vi "Read Display Values.vi"(0 "VISA resource name":refnum<visa-resource-name>, 2 "Communication Address (0)":i16 max=254 format="%x", 11 "error in (no error)":errorcluster) -> (4 "VISA resource name out":refnum<visa-resource-name>, 6 "Terminal Output Current":dbl format="%#.2g", 8 "Terminal Output Voltage":dbl format="%#.2g", 15 "error out":errorcluster)   [LabVIEW 2019, in "BK Precision 178XB Series.lvlib"]
doc: "This VI reads the voltage and current value at the terminal output of the power supply. It is the same value that is displayed on the instrument when the supply output is on."
uses:
  BK Precision 178XB Series.lvlib
panel:
  # "(c) 2009 B&K PRECISION CORPORATION.  ALL RIGHTS RESERVED."
  # "A"
  # "V"
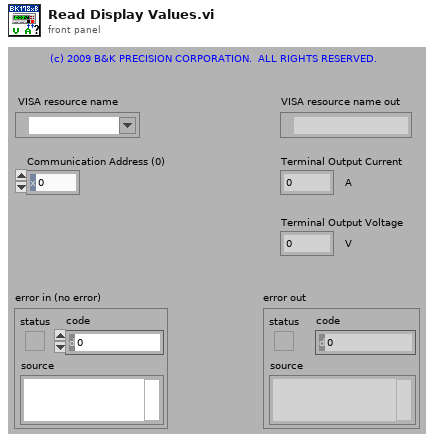
[diagram p1: front panel]
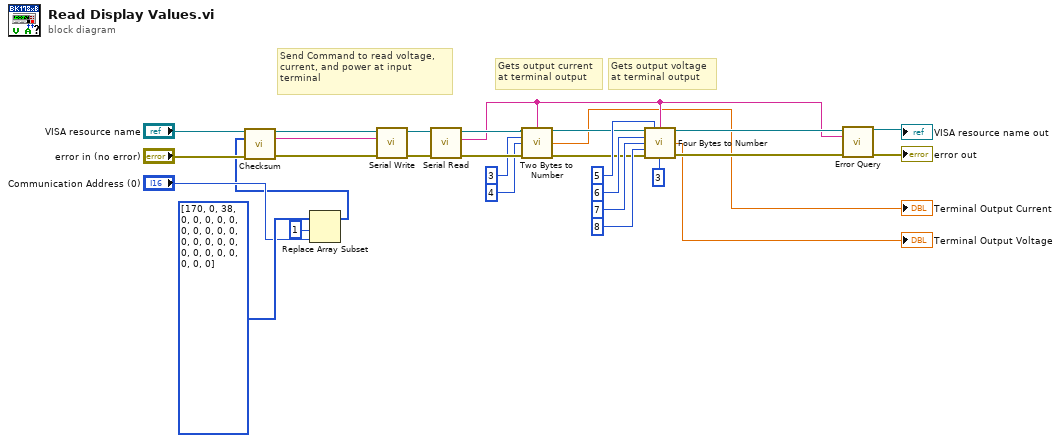
[diagram p0: block diagram]
diagram:
  # "Gets output voltage\nat terminal output"
  # "Gets output current\nat terminal output"
  # "Send Command to read voltage,\ncurrent, and power at input\nterminal"
  n1 = Replace Array Subset(array=i16[] [170, 0, 38, 0, 0, 0, 0, 0, 0, 0, 0, 0, 0, 0, 0, 0, 0, 0, 0, 0, 0, 0, 0, 0, 0, 0], new element="Communication Address (0)", index=1) -> (w1:i16[])
  n2 = call "Checksum.vi"("VISA resource name"="VISA resource name", "Command Frame Array"=w1, "error in (no error)"="error in (no error)") -> ("VISA resource name out"=w22:refnum<visa-resource-name>, "Output String"=w21:string, "error out"=w23:errorcluster)  [unwired: 8 in, 2 out]
  n3 = call "Serial Write.vi"("error in (no error)"=w23, "Input Command Frame"=w21, "VISA resource name"=w22) -> ("error out"=w27:errorcluster, "VISA resource name out"=w26:refnum<visa-resource-name>)  [unwired: 6 in, 1 out]
  n4 = call "Serial Read.vi"("error in (no error)"=w27, "VISA resource name"=w26) -> ("error out"=w16:errorcluster, "Read Buffer"=w7:string, "VISA resource name out"=w15:refnum<visa-resource-name>)  [unwired: 7 in]
  n5 = call "Two Bytes to Number.vi"("VISA resource name"=w15, "Input Command Frame"=w7, "Index 0 (3)"=3, "Index 1 (4)"=4, "error in (no error)"=w16) -> ("VISA resource name out"=w14:refnum<visa-resource-name>, "Numerical Value"=→"Terminal Output Current":dbl, "error out"=w13:errorcluster)  [unwired: 8 in]
  n6 = call "Four Bytes to Number.vi"("VISA resource name"=w14, "Index 0 (3)"=5, "Input Command Frame"=w7, "Index 1 (4)"=6, "Index 2 (5)"=7, "Index 3 (6)"=8, "error in (no error)"=w13, "Decimal Offset (3)"=3) -> ("VISA resource name out"=w8:refnum<visa-resource-name>, "Numerical Value"=→"Terminal Output Voltage":dbl, "error out"=w9:errorcluster)  [unwired: 5 in]
  n7 = call "Error Query.vi"("VISA resource name"=w8, "Input Read Buffer 1"=w7, "error in (no error)"=w9) -> ("VISA resource name out"=→"VISA resource name out":refnum<visa-resource-name>, "error out"=→"error out":errorcluster)  [unwired: 7 in, 4 out]
